vi "WRite corrected GPS.vi"(11 "Raw GPS Data":T1[](array[typedef]) {"GPS Longitude" format="%.6f"; "GPS Latitude" format="%.6f"; "Magnetic Variation (East/West)" format="%.02f [deg]"; "Date Stamp" format="%<%x>T"; "True course" format="%.02f [deg]"; "Speed in knots" format="%.02f [kts]"; "Longitude" format="%0.4f [long]"; "Latitude" format="%.04f [lat]"; "TimeStamp" format="%<%.2X>T"}) -> ()   [LabVIEW 2015, in "Log Waveform Processors.lvlib"]
uses:
  Log Waveform Processors.lvlib
  Libraries/3rd Party/NMEA_GPS/NMEA_GPRMC-data.ctl
  Libraries/3rd Party/NMEA_GPS/NMEA_LatitudeDirection.ctl
  Libraries/3rd Party/NMEA_GPS/NMEA_LongitudeDirection.ctl
  <vilib>/measure/maresamp.llb/Resample Waveform (single shot).vi
  <vilib>/Waveform/WDTFileIO.llb/Export Waveforms To Spreadsheet File (1D).vi
  GPS Instrument/GPS Instrument/GPS Instrument.lvclass
  <vilib>/measure/NI_MAPro.lvlib
  Libraries/3rd Party/NMEA_GPS/NMEA.lvlib
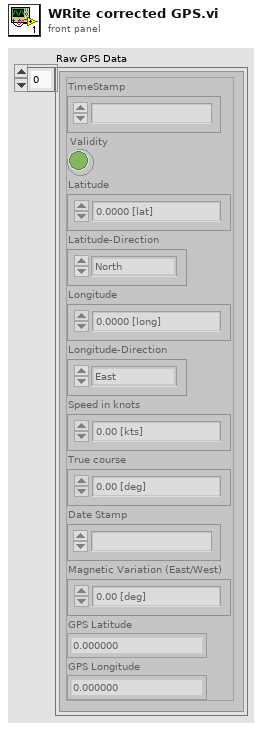
[diagram p1: front panel]
types:
  T1 = typedef "RDS Libraries.lvlib/NMEA.lvlib/NMEA_GPRMC-data.ctl" = cluster{"TimeStamp":timestamp, "Validity":bool, "Latitude":dbl, "Latitude-Direction":T2, "Longitude":dbl, "Longitude-Direction":T3, "Speed in knots":sgl, "True course":sgl, "Date Stamp":timestamp, "Magnetic Variation (East/West)":sgl, "GPS Latitude":dbl, "GPS Longitude":dbl}
  T2 = typedef "RDS Libraries.lvlib/NMEA.lvlib/NMEA_LatitudeDirection.ctl" = enum16{"", "North", "South"}
  T3 = typedef "RDS Libraries.lvlib/NMEA.lvlib/NMEA_LongitudeDirection.ctl" = enum16{"", "East", "West"}
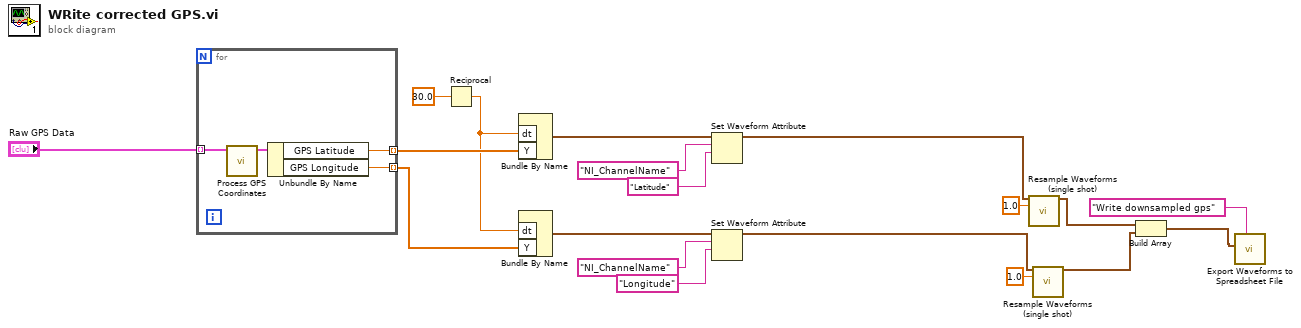
[diagram p0: block diagram]
diagram:
  n1 = for {
    tunnel: "Raw GPS Data" -> [w23] mode=indexing
    tunnel: [w21] -> w5 mode=indexing
    tunnel: [w20] -> w4 mode=indexing
    n2 = call "Process GPS Coordinates.vi"("GPRMC-data"=w23) -> ("GPRMC Data"=w22:T1)  [unwired: 10 in]
    n3 = Unbundle By Name(w22) -> ("GPS Latitude"=w21:dbl, "GPS Longitude"=w20:dbl)
  }
  n4 = Reciprocal(x=30.0) -> (1/x=w2:dbl)
  n5 = Bundle By Name("dt"=w2, "Y"=w5) -> (w16:waveform(dbl))  [unwired: 1 in]
  n6 = Bundle By Name("dt"=w2, "Y"=w4) -> (w17:waveform(dbl))  [unwired: 1 in]
  n7 = Set Waveform Attribute(5:"Latitude" ("name"), 6:"NI_ChannelName" ("name"), 7:w16) -> (3:w7:waveform(dbl))  [unwired: 1 in, 2 out]
  n8 = Set Waveform Attribute(5:"Longitude" ("name"), 6:"NI_ChannelName" ("name"), 7:w17) -> (3:w6:waveform(dbl))  [unwired: 1 in, 2 out]
  n9 = call-poly <vilib>:"Resample Waveforms (single shot).vi"("waveform in"=w7, "dt"=1.0) -> ("resampled waveform out"=w11:waveform(dbl))  [unwired: 10 in, 3 out]
  n10 = call-poly <vilib>:"Resample Waveforms (single shot).vi"("waveform in"=w6, "dt"=1.0) -> ("resampled waveform out"=w10:waveform(dbl))  [unwired: 10 in, 3 out]
  n11 = Build Array(w11, w10) -> (w9:waveform(dbl)[])
  n12 = call-poly <vilib>:"Export Waveforms to Spreadsheet File.vi"("prompt"="Write downsampled gps", "waveforms"=w9) -> ()  [unwired: 8 in, 2 out]
